vi "Hormiga_WritePort.vi"(8 "error in (no error)":errorcluster, 9 "Port Data":bool[](array[boolean]), 10 "Puerto":enum32{"PORTB", "PORTD"}(ring), 11 "VISA Refnum in":refnum<visa-resource-name>) -> (0 "error out":errorcluster, 2 "Returned Value":u8, 3 "VISA Refnum out":refnum<visa-resource-name>)   [LabVIEW 2016]
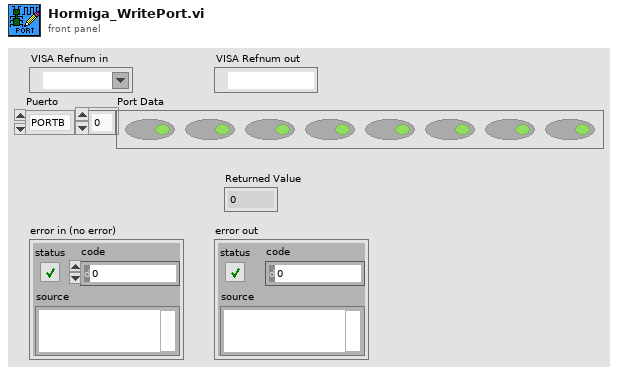
[diagram p1: front panel]
types:
  T1 = enum16{"pinMode", "digitalWrite", "digitalRead", "analogRead", "analogWrite", "PBRead", "ReadPort", "WritePort", "ReadUS", "TrisPORT"}
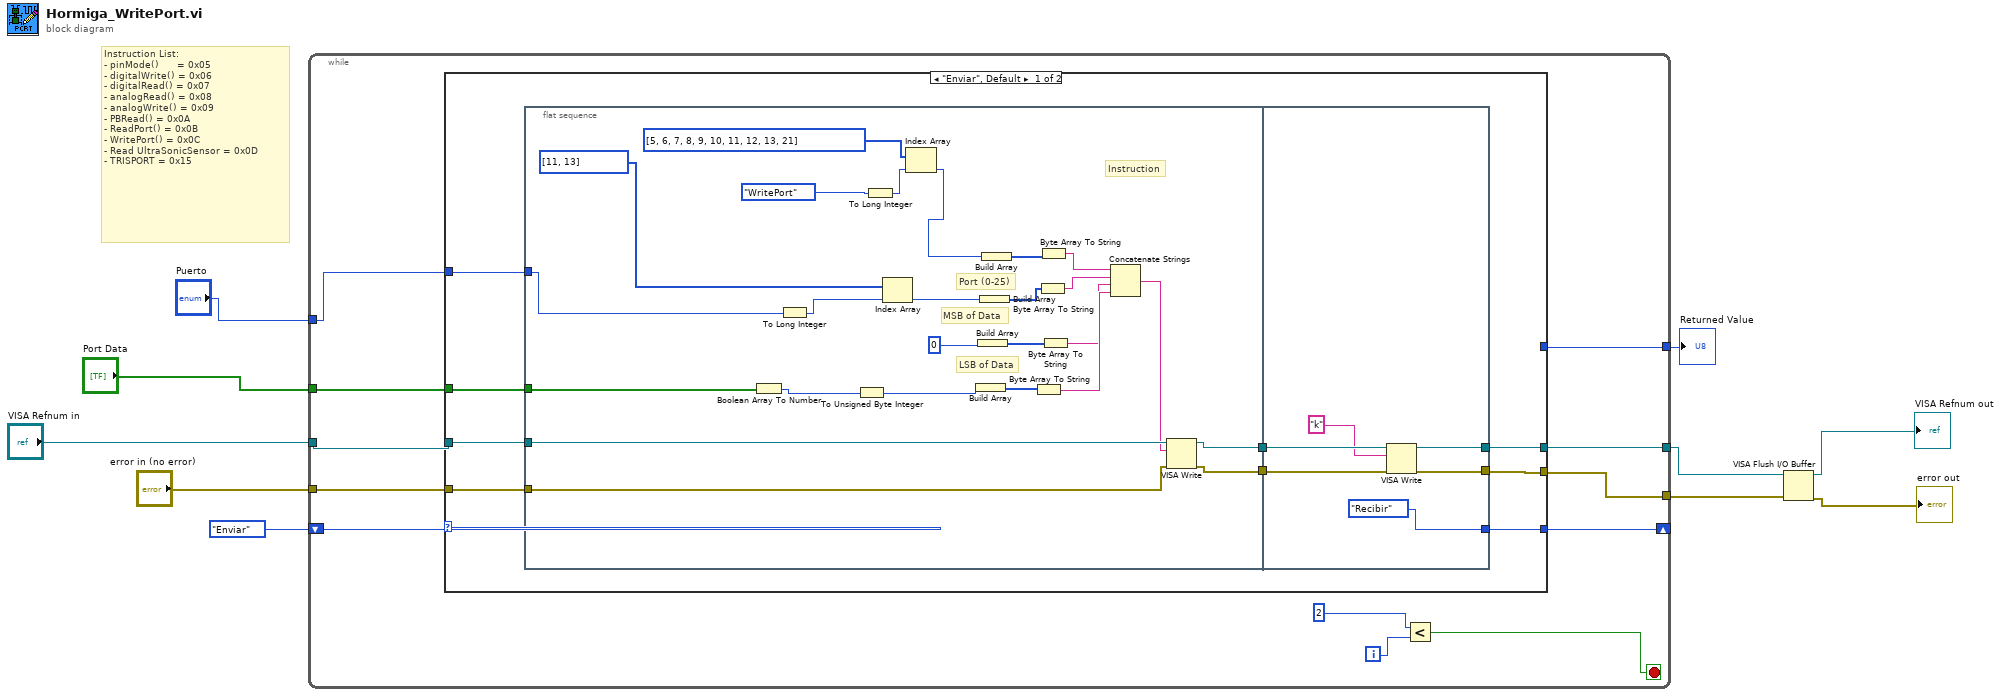
[diagram p0: block diagram]
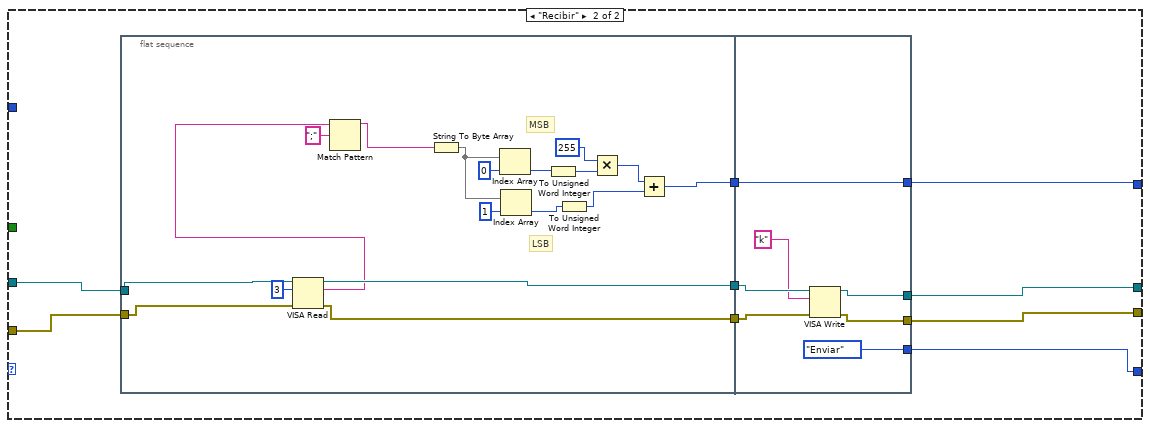
[diagram p2: hidden frame]
diagram:
  # "Instruction List:\n- pinMode()      = 0x05\n- digitalWrite() = 0x06\n- digitalRead() = 0x07\n- analogRead() = 0x08\n- analogWrite() = 0x09 \n- PBRead() = 0x0A\n- ReadPort() = 0x0B\n- WritePort() = 0x0C\n- Read UltraSonicSensor = 0x0D\n- TRISPORT = 0x15"
  n1 = while {
    shift-right: [w17] -> _
    shift-left: enum16{"Enviar", "Recibir"}."Enviar" -> [w22]
    tunnel: "error in (no error)" -> [w21]
    tunnel: "VISA Refnum in" -> [w20]
    tunnel: [w19] -> w6
    tunnel: [w18] -> w5
    tunnel: "Puerto" -> [w13]
    tunnel: [w12] -> w10
    tunnel: "Port Data" -> [w11]
    i -> [w15]
    stop <- w16 stop-if-true
    n2 = case shown="\"Enviar\", Default" w22 {
      tunnel: w21 -> [w31 w71]
      tunnel: w20 -> [w30 w70]
      tunnel: [w27 w67] -> w19
      tunnel: [w26 w66] -> w18
      tunnel: [w25 w65] -> w17
      tunnel: w13 -> [w24 _]
      tunnel: [_ w63] -> w12
      tunnel: w11 -> [w23 _]
      frame "Enviar", Default {
        n3 = flat-sequence {
          tunnel: w31 -> [w56]
          tunnel: w30 -> [w55]
          tunnel: [w54] -> w29
          tunnel: [w53] -> w28
          tunnel: w24 -> [w34]
          tunnel: w23 -> [w32]
          tunnel: w29 -> [w62]
          tunnel: w28 -> [w61]
          tunnel: [w59] -> w27
          tunnel: [w58] -> w26
          tunnel: [enum16{"Enviar", "Recibir"}."Recibir"] -> w25
          frame #0 {
            # "Instruction"
            # "LSB of Data"
            # "MSB of Data"
            # "Port (0-25)"
            n4 = Boolean Array To Number(Boolean array=w32) -> (number=w33:u32)
            n5 = To Long Integer(number=w34) -> (32bit integer=w35:i32)
            n6 = To Unsigned Byte Integer(number=w33) -> (unsigned 8bit integer=w38:u8)
            n7 = To Long Integer(number=T1."WritePort") -> (32bit integer=w41:i32)
            n8 = Index Array(array=u8[] [11, 13], index=w35) -> (element=w36:u8)
            n9 = Index Array(array=u8[] [5, 6, 7, 8, 9, 10, 11, 12, 13, 21], index=w41) -> (element=w40:u8)
            n10 = Build Array(w38) -> (w48:u8[])
            n11 = Build Array(u8 0) -> (w49:u8[])
            n12 = Build Array(w36) -> (w50:u8[])
            n13 = Build Array(w40) -> (w51:u8[])
            n14 = Byte Array To String(unsigned byte array=w48) -> (string=w47:string)
            n15 = Byte Array To String(unsigned byte array=w50) -> (string=w45:string)
            n16 = Byte Array To String(unsigned byte array=w51) -> (string=w44:string)
            n17 = Byte Array To String(unsigned byte array=w49) -> (string=w46:string)
            n18 = Concatenate Strings(w44, w45, w46, w47) -> (w39:string)
            n19 = VISA Write(VISA resource name=w55, write buffer=w39, error in (no error)=w56) -> (VISA resource name out=w53:refnum<visa-resource-name>, error out=w54:errorcluster)  [unwired: 1 out]
          }
          frame #1 {
            n20 = VISA Write(VISA resource name=w61, write buffer="k", error in (no error)=w62) -> (VISA resource name out=w58:refnum<visa-resource-name>, error out=w59:errorcluster)  [unwired: 1 out]
          }
        }
      }
      frame "Recibir" {
        n21 = flat-sequence {
          tunnel: w71 -> [w81]
          tunnel: w70 -> [w80]
          tunnel: [w89] -> w69
          tunnel: [w88] -> w68
          tunnel: [w82] -> w64
          tunnel: w69 -> [w96]
          tunnel: w68 -> [w95]
          tunnel: [w93] -> w67
          tunnel: [w92] -> w66
          tunnel: [enum16{"Enviar", "Recibir"}."Enviar"] -> w65
          tunnel: w64 -> [w90]
          tunnel: [w90] -> w63
          frame #0 {
            # "MSB"
            # "LSB"
            n22 = VISA Read(VISA resource name=w80, byte count=u32 3, error in (no error)=w81) -> (VISA resource name out=w88:refnum<visa-resource-name>, read buffer=w78:string, error out=w89:errorcluster)  [unwired: 1 out]
            n23 = Match Pattern(string=w78, regular expression=";") -> (before substring=w76:string)  [unwired: 1 in, 3 out]
            n24 = String To Byte Array(string=w76) -> (unsigned byte array=w87:u8[])
            n25 = Index Array(array=w87, index=0) -> (element=w75:u8)
            n26 = Index Array(array=w87, index=1) -> (element=w73:u8)
            n27 = To Unsigned Word Integer(number=w75) -> (unsigned 16bit integer=w74:u16)
            n28 = To Unsigned Word Integer(number=w73) -> (unsigned 16bit integer=w72:u16)
            n29 = Multiply(x=u16 255, y=w74) -> (x*y=w84:u16)
            n30 = Add(x=w84, y=w72) -> (x+y=w82:u16)
          }
          frame #1 {
            n31 = VISA Write(VISA resource name=w95, write buffer="k", error in (no error)=w96) -> (VISA resource name out=w92:refnum<visa-resource-name>, error out=w93:errorcluster)  [unwired: 1 out]
          }
        }
      }
    }
    n32 = Less?(x=2, y=w15) -> (x < y?=w16:bool)
  }
  "Returned Value" <- w10
  n33 = VISA Flush I/O Buffer(VISA resource name=w5, error in (no error)=w6) -> (VISA resource name out=→"VISA Refnum out":refnum<visa-resource-name>, error out=→"error out":errorcluster)  [unwired: 1 in]
